vi "dr_W_Q-N2.vi"(10 "Setpoint Direct":sgl min=0 max=3 step=0.1 format="%#.3g ln/min", 11 "VISA resource name\nFlow valve":refnum<visa-resource-name>="COM3") -> (0 "error out":errorcluster, 1 "Valve Output Percentage":dbl format="%#.3g %%", 2 "Measure Direct":sgl format="%#.4g ln/min", 3 "Flow-valve temperature":sgl caption="ºC" format="%#.2g ºC")   [LabVIEW 2015, in "VIPM2.lvlib"]
doc: "<b>Bronkhorst Flow Valve Driver</b>\nSets Direct Setpoint and measures temperature, flow and valve position %."
uses:
  VIPM2.lvlib
  dr Bronkhorst FLOW-BUS/Public/Configure/Setpoint/Configure Setpoint (Direct).vi
  dr Bronkhorst FLOW-BUS/Public/Data/Measure/Read Measure (Direct).vi
  dr Bronkhorst FLOW-BUS/Bronkhorst FLOW-BUS.lvlib
panel:
  # "Bronkhorst Flow Valve Driver"
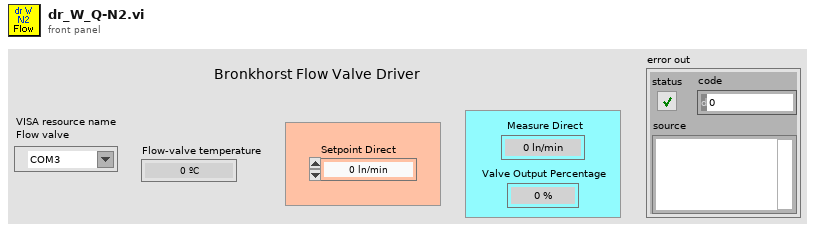
[diagram p1: front panel]
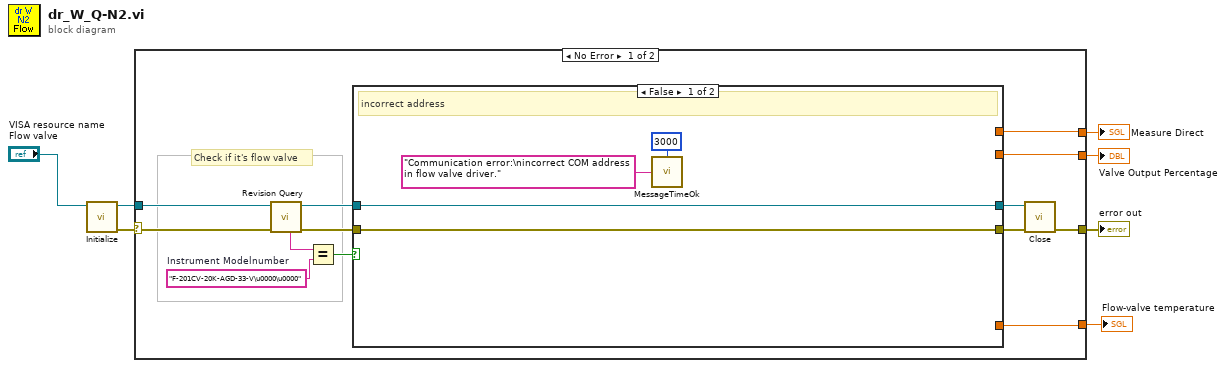
[diagram p0: block diagram]
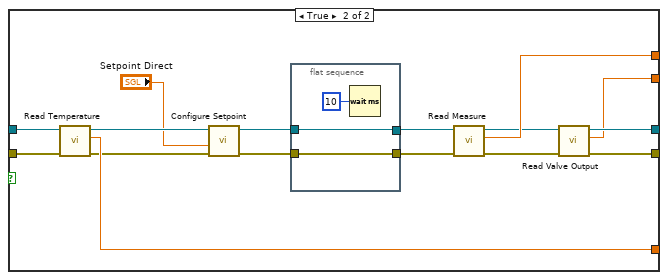
[diagram p2: hidden frame]
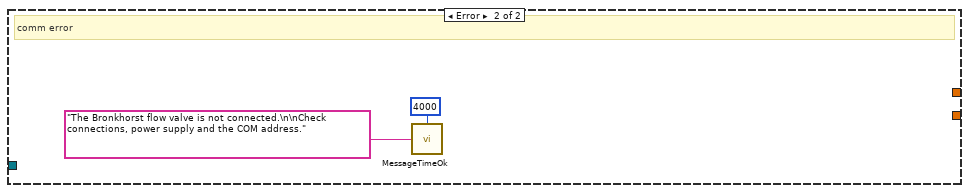
[diagram p3: hidden frame]
diagram:
  n1 = call "Initialize.vi"("VISA resource name"="VISA resource name\nFlow valve") -> ("error out"=w6:errorcluster, "VISA resource name out"=w5:refnum<visa-resource-name>)  [unwired: 9 in]
  n2 = case shown="No Error" w6 {
    selector: w6 -> [w19 _]
    tunnel: w5 -> [w20 _]
    tunnel: [w11 _] -> w4
    tunnel: [w10 _] -> w3
    tunnel: [w9 _] -> w2
    tunnel: [w8 _] -> w1
    frame No Error {
      w17 = "F-201CV-20K-AGD-33-V\u0000\u0000"  # Instrument Modelnumber
      # "Check if it's flow valve"
      n3 = call "Revision Query.vi"("error in (no error)"=w19, "VISA resource name"=w20) -> ("error out"=w14:errorcluster, "VISA resource name out"=w15:refnum<visa-resource-name>, "Instrument Modelnumber"=w18:string)  [unwired: 5 in, 2 out]
      n4 = Equal?(x=w18, y=w17) -> (x = y?=w16:bool)
      n5 = case shown="False" w16 {
        tunnel: w15 -> [w23 w40]
        tunnel: w14 -> [w24 w39]
        tunnel: [w24 w26] -> w12
        tunnel: [w23 w27] -> w13
        tunnel: [_ w38] -> w11
        tunnel: [_ w30] -> w9
        tunnel: [_ w25] -> w8
        frame False {
          # "incorrect address"
          n6 = call "MessageTimeOk.vi"("time (ms)"=3000, "missage"="Communication error:\nincorrect COM address in flow valve driver.") -> ()  [unwired: 4 in]
        }
        frame True {
          n7 = call "Read Temperature.vi"("error in (no error)"=w39, "VISA resource name"=w40) -> ("error out"=w36:errorcluster, "Temperature (deg C)"=w38:sgl, "VISA resource name out"=w37:refnum<visa-resource-name>)  [unwired: 7 in]
          n8 = call-poly "Configure Setpoint.vi"("error in (no error)"=w36, "Setpoint Direct (0)"="Setpoint Direct", "VISA resource name"=w37) -> ("error out"=w33:errorcluster, "VISA resource name out"=w34:refnum<visa-resource-name>)  [unwired: 7 in]
          n9 = flat-sequence {
            tunnel: [w43] -> w32
            tunnel: w34 -> [w43]
            tunnel: [w42] -> w31
            tunnel: w33 -> [w42]
            frame #0 {
              n10 = Wait (ms)(milliseconds to wait=u32 10) -> ()  [unwired: 1 out]
            }
          }
          n11 = call-poly "Read Measure.vi"("error in (no error)"=w31, "VISA resource name"=w32) -> ("error out"=w28:errorcluster, "Measure Direct"=w30:sgl, "VISA resource name out"=w29:refnum<visa-resource-name>)  [unwired: 7 in]
          n12 = call "Read Valve Output.vi"("error in (no error)"=w28, "VISA resource name"=w29) -> ("error out"=w26:errorcluster, "Valve Output Percentage"=w25:dbl, "VISA resource name out"=w27:refnum<visa-resource-name>)  [unwired: 6 in, 1 out]
        }
      }
      n13 = call "Close.vi"("error in (no error)"=w12, "VISA resource name"=w13) -> ("error out"=w10:errorcluster)  [unwired: 9 in]
    }
    frame Error {
      # "comm error"
      n14 = call "MessageTimeOk.vi"("time (ms)"=4000, "missage"="The Bronkhorst flow valve is not connected.\n\nCheck connections, power supply and the COM address.") -> ()  [unwired: 4 in]
    }
  }
  "Flow-valve temperature" <- w4
  "error out" <- w3
  "Measure Direct" <- w2
  "Valve Output Percentage" <- w1
